vi "Query Chan Parameters (Output).vi"(7 "Channel (1: Chan A)":i32(ring)=1 items=["Channel A"=1, "Channel B"=2, "Channel C"=3, "Channel D"=4, "Channel E"=5, "Channel F"=6, "Channel G"=7, "Channel H"=8], 8 "error in (no error)":errorcluster, 11 "VISA resource name":refnum<visa-resource-name>) -> (0 "error out":errorcluster, 2 "Output Parameters":T1={"Polarity Out"=FALSE, "Level Value"=nan, "Level Out"=enum."TTL", "MUX Value"=0} {"Level Value" format="%.3p"}, 3 "VISA resource name out":refnum<visa-resource-name>)   [LabVIEW 2012, in "Quantum Composers 9000 Series.lvlib"]
doc: "This VI is used to read the output configuration of the selected channel."
uses:
  Quantum Composers 9000 Series.lvlib
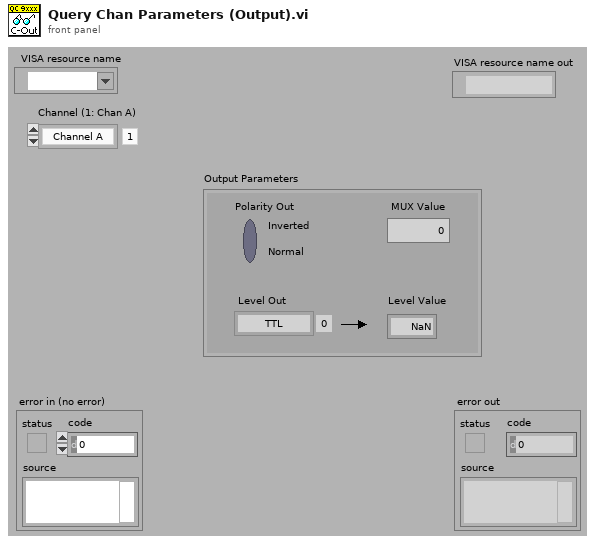
[diagram p1: front panel]
types:
  T1 = cluster{"Polarity Out":bool, "Level Value":dbl, "Level Out":enum16{"TTL", "Adjustable", "35 Volt", "Optical"}, "MUX Value":i32}
  T2 = enum16{"TTL", "Adjustable", "35 Volt", "Optical"}
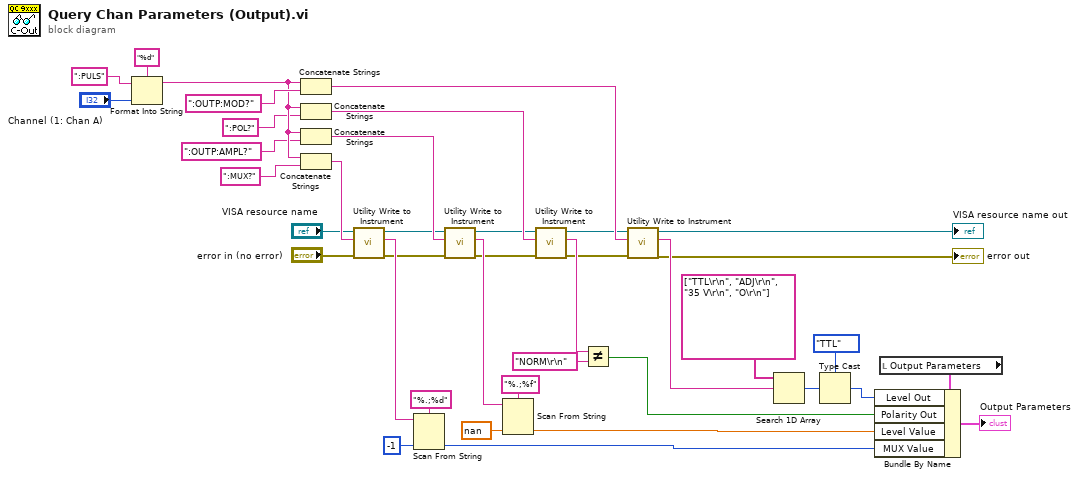
[diagram p0: block diagram]
diagram:
  n1 = Format Into String(format string="%d", initial string=":PULS", "Channel (1: Chan A)") -> (resulting string=w32:string)  [unwired: 1 in, 1 out]
  n2 = Concatenate Strings(w32, ":OUTP:MOD?") -> (w25:string)
  n3 = Concatenate Strings(w32, ":POL?") -> (w26:string)
  n4 = Concatenate Strings(w32, ":OUTP:AMPL?") -> (w27:string)
  n5 = Concatenate Strings(w32, ":MUX?") -> (w28:string)
  n6 = call "Utility Write to Instrument.vi"("error in (no error)"="error in (no error)", "Write Buffer"=w28, "VISA resource name"="VISA resource name") -> ("error out"=w22:errorcluster, "Read Buffer"=w37:string, "VISA resource name out"=w21:refnum<visa-resource-name>)  [unwired: 6 in]
  n7 = Scan From String(format string="%.;%d", input string=w37, default 1=-1 ("default value 1")) -> (output 1=w8:i32)  [unwired: 2 in, 3 out]
  n8 = call "Utility Write to Instrument.vi"("error in (no error)"=w22, "Write Buffer"=w27, "VISA resource name"=w21) -> ("error out"=w13:errorcluster, "Read Buffer"=w20:string, "VISA resource name out"=w12:refnum<visa-resource-name>)  [unwired: 6 in]
  n9 = Scan From String(format string="%.;%f", input string=w20, default 1=nan ("default value 1")) -> (output 1=w6:dbl)  [unwired: 2 in, 3 out]
  n10 = call "Utility Write to Instrument.vi"("error in (no error)"=w13, "Write Buffer"=w26, "VISA resource name"=w12) -> ("error out"=w14:errorcluster, "Read Buffer"=w18:string, "VISA resource name out"=w15:refnum<visa-resource-name>)  [unwired: 6 in]
  n11 = Not Equal?(x=w18, y="NORM\r\n") -> (x != y?=w7:bool)
  n12 = call "Utility Write to Instrument.vi"("error in (no error)"=w14, "Write Buffer"=w25, "VISA resource name"=w15) -> ("error out"=→"error out":errorcluster, "Read Buffer"=w16:string, "VISA resource name out"=→"VISA resource name out":refnum<visa-resource-name>)  [unwired: 6 in]
  n13 = Search 1D Array(1D array=string[] ["TTL\r\n", "ADJ\r\n", "35 V\r\n", "O\r\n"], element=w16) -> (index of element=w3:i32)  [unwired: 1 in]
  n14 = Type Cast(type=T2."TTL" ("Level Out"), x=w3) -> (*(type *) &x=w1:T2)
  n15 = local read "Output Parameters"() -> (w4:T1)
  n16 = Bundle By Name(cluster=w4, "Level Out"=w1, "Polarity Out"=w7, "Level Value"=w6, "MUX Value"=w8) -> (→"Output Parameters":T1)
